vi "CSM - Load Configuration Variables From File.vi"(5 "Section Postfix (\"\")":string, 8 "error in (no error)":errorcluster, 9 "Configuration Path":path) -> (2 "error out":errorcluster)   [LabVIEW 2017, in "INI-Static-Variable-Support.lvlib"]
uses:
  INI-Static-Variable-Support.lvlib
  _Support/_fgv-oper.ctl
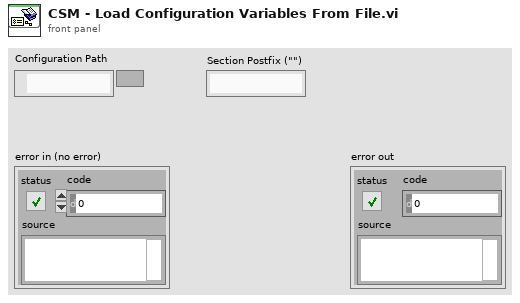
[diagram p1: front panel]
types:
  T1 = typedef "INI-Static-Variable-Support.lvlib/_fgv-oper.ctl" = enum16{"Read", "Write", "Sync", "Sessions", "List Keys", "Load", "List Files", "List Variables", "List Permanent Variables", "Mark Temp Variable as Permenent", "unload", "INIConfig(Memory)", "Reset", "Restore Variable Value"}
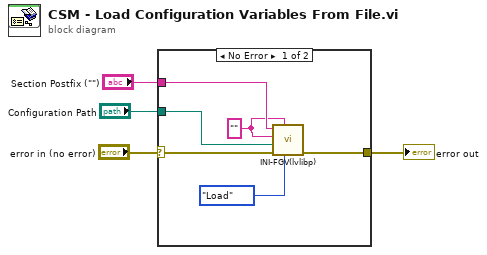
[diagram p0: block diagram]
diagram:
  n1 = case shown="No Error" "error in (no error)" {
    selector: "error in (no error)" -> [w8 w11]
    tunnel: "Configuration Path" -> [w9 _]
    tunnel: [w7 w11] -> w2
    tunnel: "Section Postfix (\"\")" -> [w6 _]
    frame No Error {
      w5 = "" (">> Variable Name >>")
      n2 = call "INI-FGV(lvlibp).vi"("Enum"=_fgv-oper."Load", "Prefered Section"=w5, "error IN"=w8, "Path"=w9, ">> Default Value >>"=w5, ">> Variable Name >>"=w6) -> ("error out"=w7:errorcluster)  [unwired: 2 in, 3 out]
    }
    frame Error {
    }
  }
  "error out" <- w2
